vi "Get Max Range.vi"(8 "error in (no error)":errorcluster, 10 "Max Range In":T2, 11 "Plot Representation In":T1) -> (0 "error out":errorcluster, 2 "Max Range Out":T2, 3 "Plot Representation Out":T1)   [LabVIEW 2017, in "3D Plot Datatype.lvclass"]
uses:
  <vilib>/Math Plots/3D Math Plots/3D Plot/3D Plot Datatype/3D Plot Datatype.lvclass
  <vilib>/Math Plots/3D Math Plots/3D Plot/3D Plot/Typedef/Range Clusters.ctl
  <vilib>/Math Plots/3D Math Plots/3D Plot/3D Plot/Typedef/Plot Representation.ctl
  <vilib>/Math Plots/3D Math Plots/3D Plot/3D Plot/Typedef/Mesh Data.ctl
  <vilib>/Math Plots/3D Math Plots/3D Plot/3D Plot/3D Plot.lvclass
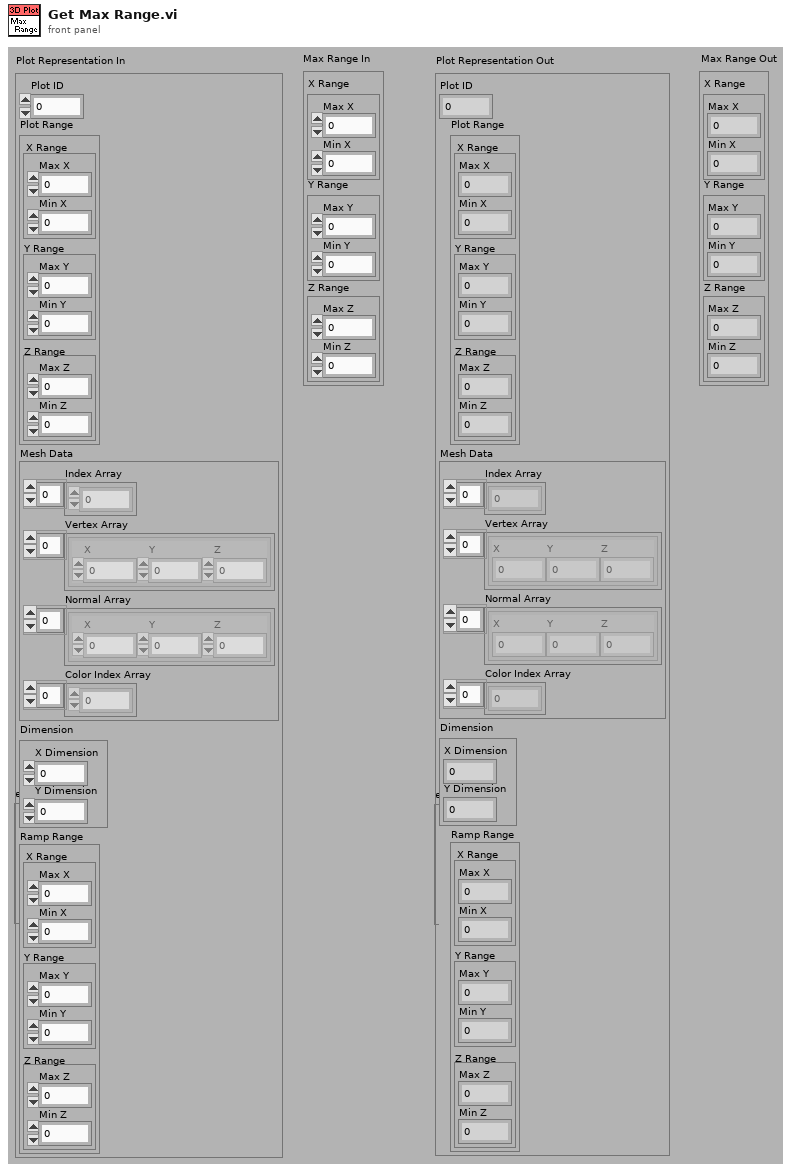
[diagram p1: front panel]
types:
  T1 = typedef "3D Plot.lvclass/Plot Representation.ctl" = cluster{"Plot ID":i32, "Plot Range":T2, "Mesh Data":T3, "Dimension":cluster{"X Dimension":i32, "Y Dimension":i32}, "Ramp Range":T2}
  T2 = typedef "3D Plot.lvclass/Range Clusters.ctl" = cluster{"X Range":cluster{"Max X":sgl, "Min X":sgl}, "Y Range":cluster{"Max Y":sgl, "Min Y":sgl}, "Z Range":cluster{"Max Z":sgl, "Min Z":sgl}}
  T3 = typedef "3D Plot.lvclass/Mesh Data.ctl" = cluster{"Index Array":u32[], "Vertex Array":cluster{"X":sgl, "Y":sgl, "Z":sgl}[], "Normal Array":cluster{"X":sgl, "Y":sgl, "Z":sgl}[], "Color Index Array":i32[]}
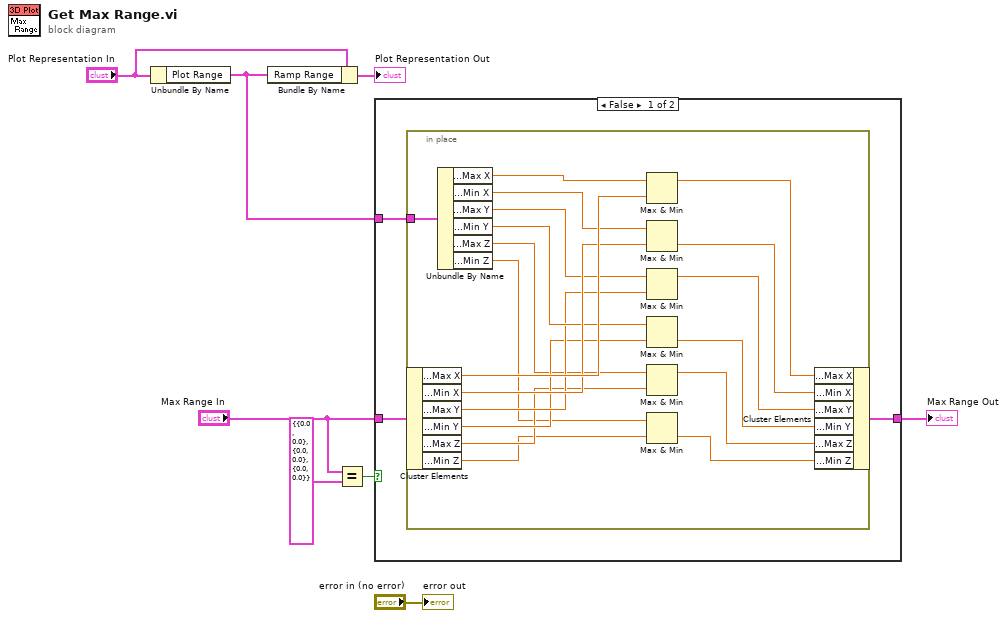
[diagram p0: block diagram]
diagram:
  n1 = Unbundle By Name("Plot Representation In") -> ("Plot Range"=w2:T2)
  n2 = Bundle By Name(cluster="Plot Representation In", "Ramp Range"=w2) -> (→"Plot Representation Out":T1)
  n3 = Equal?(x="Max Range In", y=T2 {"X Range"={"Max X"=0.0, "Min X"=0.0}, "Y Range"={"Max Y"=0.0, "Min Y"=0.0}, "Z Range"={"Max Z"=0.0, "Min Z"=0.0}} ("Max Range In")) -> (x = y?=w7:bool)
  n4 = case shown="False" w7 {
    tunnel: "Max Range In" -> [w11 _]
    tunnel: w2 -> [w10 w31]
    tunnel: [w9 w31] -> w1
    frame False {
      n5 = in-place {
        in-place-border: w10 -> [w12]
        n6 = in-place-cluster #1(w11) -> ("X Range.Max X"=w29:sgl, "X Range.Min X"=w26:sgl, "Y Range.Max Y"=w20:sgl, "Y Range.Min Y"=w19:sgl, "Z Range.Max Z"=w17:sgl, "Z Range.Min Z"=w14:sgl)
        n7 = Unbundle By Name(w12) -> ("X Range.Max X"=w30:sgl, "X Range.Min X"=w27:sgl, "Y Range.Max Y"=w21:sgl, "Y Range.Min Y"=w22:sgl, "Z Range.Max Z"=w18:sgl, "Z Range.Min Z"=w13:sgl)
        n8 = Max & Min(x=w30, y=w29) -> (max(x,y)=w28:sgl)  [unwired: 1 out]
        n9 = Max & Min(x=w27, y=w26) -> (min(x,y)=w25:sgl)  [unwired: 1 out]
        n10 = Max & Min(x=w21, y=w20) -> (max(x,y)=w24:sgl)  [unwired: 1 out]
        n11 = Max & Min(x=w22, y=w19) -> (min(x,y)=w23:sgl)  [unwired: 1 out]
        n12 = Max & Min(x=w18, y=w17) -> (max(x,y)=w16:sgl)  [unwired: 1 out]
        n13 = Max & Min(x=w13, y=w14) -> (min(x,y)=w15:sgl)  [unwired: 1 out]
        n14 = in-place-cluster #1("X Range.Max X"=w28, "X Range.Min X"=w25, "Y Range.Max Y"=w24, "Y Range.Min Y"=w23, "Z Range.Max Z"=w16, "Z Range.Min Z"=w15) -> (w9:T2)
      }
    }
    frame True {
    }
  }
  "Max Range Out" <- w1
  "error out" <- "error in (no error)"
